vi "save AutoCad cmds.vi"(7 "DesignRequest":T1, 10 "error in":errorcluster, 11 "MathCAD results":T2) -> (2 "error out":errorcluster)   [LabVIEW 2015]
uses:
  Variable cluster.ctl
  Design Request.ctl
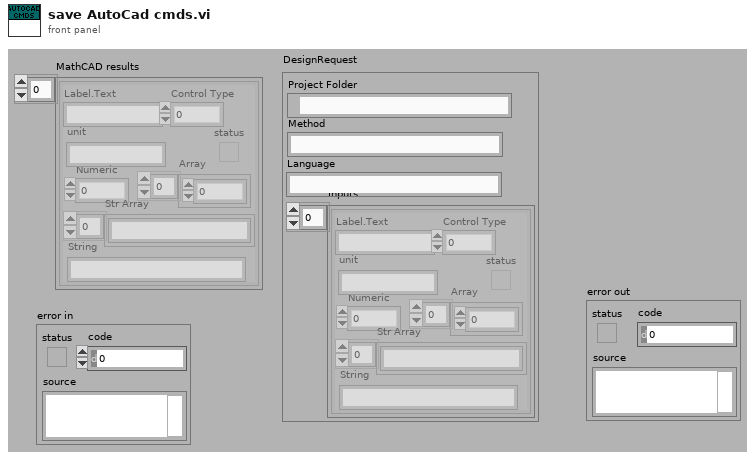
[diagram p1: front panel]
types:
  T1 = typedef "Design Request.ctl" = cluster{"Project Folder":path, "Method":string, "Inputs":T2, "Language":string}
  T2 = typedef "Variable cluster.ctl" = cluster{"Label.Text":string, "Control Type":u32, "Numeric":dbl, "Array":dbl[], "status":bool, "Str Array":string[], "String":string, "unit":string}[]
  T3 = enum16{"open", "replace", "create", "open or create", "replace or create", "replace or create with confirmation"}
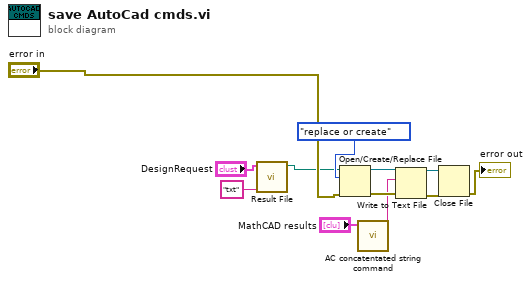
[diagram p0: block diagram]
diagram:
  n1 = call "Result File.vi"("File Type"="txt", "DesignRequest"="DesignRequest") -> ("File path"=w1:path)  [unwired: 8 in, 1 out]
  n2 = Open/Create/Replace File(file path (use dialog)=w1, error in="error in", operation (0:open)=T3."replace or create") -> (refnum out=w9:refnum<file>, error out=w8:errorcluster)  [unwired: 3 in, 1 out]
  n3 = call "AC concatentated string command.vi"("MathCAD results"="MathCAD results") -> ("AC concatenated string"=w7:string)  [unwired: 10 in]
  n4 = Write to Text File(file (use dialog)=w9, text=w7, error in=w8) -> (refnum out=w10:refnum<file>, error out=w11:errorcluster)  [unwired: 1 in, 1 out]
  n5 = Close File(refnum=w10, error in=w11) -> (error out=→"error out":errorcluster)  [unwired: 1 out]
